vi "Cowl_Hardware_Begin.vi"(8 "error in":errorcluster) -> (0 "error out":errorcluster)   [LabVIEW 2020]
uses:
  <vilib>/Rock Robotics/WPI/ThirdParty/Phoenix-LabVIEW/Motor Controller/Controls/CTRE_Phoenix_MotorControl_NeutralMode.ctl
  <vilib>/Rock Robotics/WPI/ThirdParty/Phoenix-LabVIEW/Motor Controller/Controls/CTRE_Phoenix_MotorControl_SupplyCurrentLimitConfiguration.ctl
  Cowl_Hardware_Globals.vi
  <vilib>/Rock Robotics/WPI/ThirdParty/Phoenix-LabVIEW/Motor Controller/Controls/CTRE_Phoenix_MotorControl_StatusFrameEnhanced.ctl
panel:
  out "appended array":u32[](array[numeric])
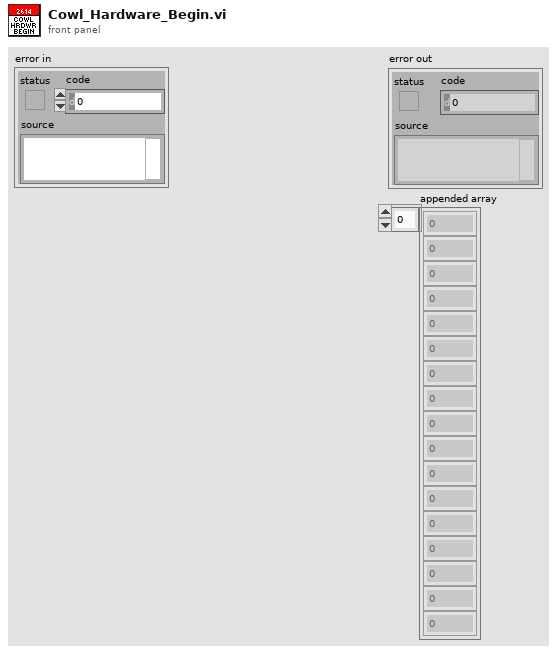
[diagram p1: front panel]
types:
  T1 = typedef "CTRE_Phoenix_MotorControl_SupplyCurrentLimitConfiguration.ctl" = cluster{"Enable?":bool, "Current Limit":dbl, "Threshold Current":dbl, "Threshold Time":dbl}
  T2 = typedef "CTRE_Phoenix_MotorControl_NeutralMode.ctl" = enum8{"EEPROMSetting", "Override to Coast", "Override to Brake"}
  T3 = typedef "WPI_MotorControlDeviceRef.ctl" = cluster{"DeviceStatus":errorcluster, "Type":T4, "PWM":cluster{"PWM Channel":T5, "DeadBand":T6}, "CAN":cluster{"Device Number":u8, "SetOutput VI Ref":variant, "GetOutput VI Ref":variant, "Enable VI Ref":variant, "Disable VI Ref":variant, "Data":variant}, "Invert":bool, "DIO PWM":cluster{"PWM \"Enable\" Channel":T5, "DIOChannel":T7, "PWM Rate":dbl}}
  T4 = typedef "WPI_MotorControlType.ctl" = enum16{"PWM", "CAN", "DIO PWM"}
  T5 = typedef "FPGA_DIOPWMChannel.ctl" = enum8{"PWM 0", "PWM 1", "PWM 2", "PWM 3", "PWM 4", "PWM 5", "PWM 6", "PWM 7", "PWM 8", "PWM 9", "PWM MXP 0", "PWM MXP 1", "PWM MXP 2", "PWM MXP 3", "PWM MXP 4", "PWM MXP 5", "PWM MXP 6", "PWM MXP 7", "PWM MXP 8", "PWM MXP 9", "Invalid"}
  T6 = typedef "WPI_PWMDeadband.ctl" = cluster{"Name":string, "maxPositivePwm":i32, "minPositivePwm":i32, "centerPwm":i32, "maxNegativePwm":i32, "minNegativePwm":i32, "angularRange":u16}
  T7 = typedef "FPGA_DIOChannel.ctl" = enum8{"DIO 0", "DIO 1", "DIO 2", "DIO 3", "DIO 4", "DIO 5", "DIO 6", "DIO 7", "DIO 8", "DIO 9", "DIO MXP 0", "DIO MXP 1", "DIO MXP 2", "DIO MXP 3", "DIO MXP 4", "DIO MXP 5", "DIO MXP 6", "DIO MXP 7", "DIO MXP 8", "DIO MXP 9", "DIO MXP 10", "DIO MXP 11", "DIO MXP 12", "DIO MXP 13", "DIO MXP 14", "DIO MXP 15", "SPI Port CS1", "SPI Port CS2", "SPI Port CS3", "SPI Port MISO", "SPI Port MOSI", "Invalid"}
  T8 = typedef "CTRE_Phoenix_MotorControl_StatusFrameEnhanced.ctl" = u16
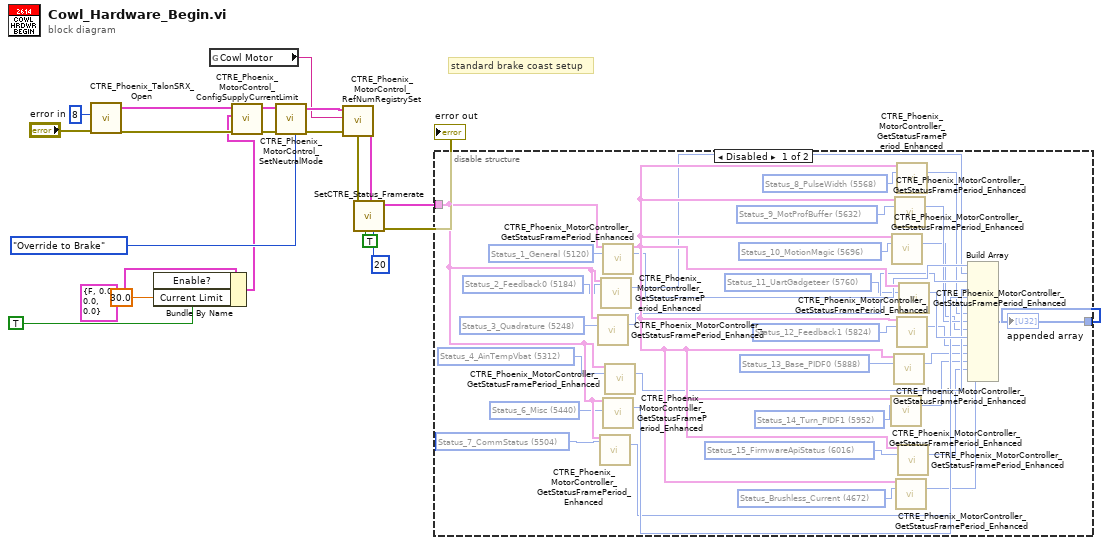
[diagram p0: block diagram]
diagram:
  # "standard brake coast setup"
  n1 = call <vilib>:"CTRE_Phoenix_TalonSRX_Open.vi"("error in"="error in", "Device Number"=u8 8) -> ("error out"=w17:errorcluster, "PhoenixMotorControlDevRef"=w18:T3)  [unwired: 8 in]
  n2 = Bundle By Name(cluster=T1 {"Enable?"=FALSE, "Current Limit"=0.0, "Threshold Current"=0.0, "Threshold Time"=0.0} ("Supply Current Limit Configuration"), "Enable?"=TRUE, "Current Limit"=30.0) -> (w10:T1)
  n3 = global read "Cowl_Hardware_Globals.vi" "Cowl Motor"() -> (w9:string)
  n4 = call <vilib>:"CTRE_Phoenix_MotorControl_ConfigSupplyCurrentLimit.vi"("error in (no error)"=w17, "Supply Current Limit Configuration"=w10, "PhoenixMotorControlDevRef"=w18) -> ("error out"=w16:errorcluster, "PhoenixMotorControlDevRef"=w15:T3)  [unwired: 7 in]
  n5 = call <vilib>:"CTRE_Phoenix_MotorControl_SetNeutralMode.vi"("error in (no error)"=w16, "Motor Control Neutral Mode"=CTRE_Phoenix_MotorControl_NeutralMode."Override to Brake", "PhoenixMotorControlDevRef"=w15) -> ("error out"=w14:errorcluster, "PhoenixMotorControlDevRef"=w19:T3)  [unwired: 7 in]
  n6 = call <vilib>:"CTRE_Phoenix_MotorControl_RefNumRegistrySet.vi"("error in (no error)"=w14, "refnum name"=w9, "PhoenixMotorControlDevRef"=w19) -> ("error out"=w6:errorcluster, "PhoenixMotorControlDevRef"=w7:T3)  [unwired: 7 in]
  n7 = call "SetCTRE_Status_Framerate.vi"("STATUS2Override(ms)"=20, "STATUS2OutsideOverride"=TRUE, "error in (no error)"=w6, "PhoenixMotorControlDevRef"=w7) -> ("error out"=→"error out":errorcluster, "PhoenixMotorControlDevRef 2"=w1:T3)  [unwired: 6 in]
  n8 = disable-structure shown="Disabled" {
    disable-tunnel: w1 -> [w50 _]
    disable-tunnel: [w54 _] -> w2
    frame Disabled {
      w22 = T8 5760 items=["Status_1_General"=5120, "Status_2_Feedback0"=5184, "Status_3_Quadrature"=5248, "Status_4_AinTempVbat"=5312, "Status_6_Misc"=5440, "Status_7_CommStatus"=5504, "Status_8_PulseWidth"=5568, "Status_9_MotProfBuffer"=5632, "Status_10_MotionMagic"=5696, "Status_11_UartGadgeteer"=5760, "Status_12_Feedback1"=5824, "Status_13_Base_PIDF0"=5888, "Status_14_Turn_PIDF1"=5952, "Status_15_FirmwareApiStatus"=6016, "Status_Brushless_Current"=4672] ("Status Frame")
      w23 = T8 5696 items=["Status_1_General"=5120, "Status_2_Feedback0"=5184, "Status_3_Quadrature"=5248, "Status_4_AinTempVbat"=5312, "Status_6_Misc"=5440, "Status_7_CommStatus"=5504, "Status_8_PulseWidth"=5568, "Status_9_MotProfBuffer"=5632, "Status_10_MotionMagic"=5696, "Status_11_UartGadgeteer"=5760, "Status_12_Feedback1"=5824, "Status_13_Base_PIDF0"=5888, "Status_14_Turn_PIDF1"=5952, "Status_15_FirmwareApiStatus"=6016, "Status_Brushless_Current"=4672] ("Status Frame")
      w25 = T8 5888 items=["Status_1_General"=5120, "Status_2_Feedback0"=5184, "Status_3_Quadrature"=5248, "Status_4_AinTempVbat"=5312, "Status_6_Misc"=5440, "Status_7_CommStatus"=5504, "Status_8_PulseWidth"=5568, "Status_9_MotProfBuffer"=5632, "Status_10_MotionMagic"=5696, "Status_11_UartGadgeteer"=5760, "Status_12_Feedback1"=5824, "Status_13_Base_PIDF0"=5888, "Status_14_Turn_PIDF1"=5952, "Status_15_FirmwareApiStatus"=6016, "Status_Brushless_Current"=4672] ("Status Frame")
      w27 = T8 6016 items=["Status_1_General"=5120, "Status_2_Feedback0"=5184, "Status_3_Quadrature"=5248, "Status_4_AinTempVbat"=5312, "Status_6_Misc"=5440, "Status_7_CommStatus"=5504, "Status_8_PulseWidth"=5568, "Status_9_MotProfBuffer"=5632, "Status_10_MotionMagic"=5696, "Status_11_UartGadgeteer"=5760, "Status_12_Feedback1"=5824, "Status_13_Base_PIDF0"=5888, "Status_14_Turn_PIDF1"=5952, "Status_15_FirmwareApiStatus"=6016, "Status_Brushless_Current"=4672] ("Status Frame")
      w29 = T8 5952 items=["Status_1_General"=5120, "Status_2_Feedback0"=5184, "Status_3_Quadrature"=5248, "Status_4_AinTempVbat"=5312, "Status_6_Misc"=5440, "Status_7_CommStatus"=5504, "Status_8_PulseWidth"=5568, "Status_9_MotProfBuffer"=5632, "Status_10_MotionMagic"=5696, "Status_11_UartGadgeteer"=5760, "Status_12_Feedback1"=5824, "Status_13_Base_PIDF0"=5888, "Status_14_Turn_PIDF1"=5952, "Status_15_FirmwareApiStatus"=6016, "Status_Brushless_Current"=4672] ("Status Frame")
      w31 = T8 5568 items=["Status_1_General"=5120, "Status_2_Feedback0"=5184, "Status_3_Quadrature"=5248, "Status_4_AinTempVbat"=5312, "Status_6_Misc"=5440, "Status_7_CommStatus"=5504, "Status_8_PulseWidth"=5568, "Status_9_MotProfBuffer"=5632, "Status_10_MotionMagic"=5696, "Status_11_UartGadgeteer"=5760, "Status_12_Feedback1"=5824, "Status_13_Base_PIDF0"=5888, "Status_14_Turn_PIDF1"=5952, "Status_15_FirmwareApiStatus"=6016, "Status_Brushless_Current"=4672] ("Status Frame")
      w33 = T8 4672 items=["Status_1_General"=5120, "Status_2_Feedback0"=5184, "Status_3_Quadrature"=5248, "Status_4_AinTempVbat"=5312, "Status_6_Misc"=5440, "Status_7_CommStatus"=5504, "Status_8_PulseWidth"=5568, "Status_9_MotProfBuffer"=5632, "Status_10_MotionMagic"=5696, "Status_11_UartGadgeteer"=5760, "Status_12_Feedback1"=5824, "Status_13_Base_PIDF0"=5888, "Status_14_Turn_PIDF1"=5952, "Status_15_FirmwareApiStatus"=6016, "Status_Brushless_Current"=4672] ("Status Frame")
      w35 = T8 5824 items=["Status_1_General"=5120, "Status_2_Feedback0"=5184, "Status_3_Quadrature"=5248, "Status_4_AinTempVbat"=5312, "Status_6_Misc"=5440, "Status_7_CommStatus"=5504, "Status_8_PulseWidth"=5568, "Status_9_MotProfBuffer"=5632, "Status_10_MotionMagic"=5696, "Status_11_UartGadgeteer"=5760, "Status_12_Feedback1"=5824, "Status_13_Base_PIDF0"=5888, "Status_14_Turn_PIDF1"=5952, "Status_15_FirmwareApiStatus"=6016, "Status_Brushless_Current"=4672] ("Status Frame")
      w37 = T8 5632 items=["Status_1_General"=5120, "Status_2_Feedback0"=5184, "Status_3_Quadrature"=5248, "Status_4_AinTempVbat"=5312, "Status_6_Misc"=5440, "Status_7_CommStatus"=5504, "Status_8_PulseWidth"=5568, "Status_9_MotProfBuffer"=5632, "Status_10_MotionMagic"=5696, "Status_11_UartGadgeteer"=5760, "Status_12_Feedback1"=5824, "Status_13_Base_PIDF0"=5888, "Status_14_Turn_PIDF1"=5952, "Status_15_FirmwareApiStatus"=6016, "Status_Brushless_Current"=4672] ("Status Frame")
      w39 = T8 5120 items=["Status_1_General"=5120, "Status_2_Feedback0"=5184, "Status_3_Quadrature"=5248, "Status_4_AinTempVbat"=5312, "Status_6_Misc"=5440, "Status_7_CommStatus"=5504, "Status_8_PulseWidth"=5568, "Status_9_MotProfBuffer"=5632, "Status_10_MotionMagic"=5696, "Status_11_UartGadgeteer"=5760, "Status_12_Feedback1"=5824, "Status_13_Base_PIDF0"=5888, "Status_14_Turn_PIDF1"=5952, "Status_15_FirmwareApiStatus"=6016, "Status_Brushless_Current"=4672] ("Status Frame")
      w40 = T8 5504 items=["Status_1_General"=5120, "Status_2_Feedback0"=5184, "Status_3_Quadrature"=5248, "Status_4_AinTempVbat"=5312, "Status_6_Misc"=5440, "Status_7_CommStatus"=5504, "Status_8_PulseWidth"=5568, "Status_9_MotProfBuffer"=5632, "Status_10_MotionMagic"=5696, "Status_11_UartGadgeteer"=5760, "Status_12_Feedback1"=5824, "Status_13_Base_PIDF0"=5888, "Status_14_Turn_PIDF1"=5952, "Status_15_FirmwareApiStatus"=6016, "Status_Brushless_Current"=4672] ("Status Frame")
      w42 = T8 5184 items=["Status_1_General"=5120, "Status_2_Feedback0"=5184, "Status_3_Quadrature"=5248, "Status_4_AinTempVbat"=5312, "Status_6_Misc"=5440, "Status_7_CommStatus"=5504, "Status_8_PulseWidth"=5568, "Status_9_MotProfBuffer"=5632, "Status_10_MotionMagic"=5696, "Status_11_UartGadgeteer"=5760, "Status_12_Feedback1"=5824, "Status_13_Base_PIDF0"=5888, "Status_14_Turn_PIDF1"=5952, "Status_15_FirmwareApiStatus"=6016, "Status_Brushless_Current"=4672] ("Status Frame")
      w44 = T8 5440 items=["Status_1_General"=5120, "Status_2_Feedback0"=5184, "Status_3_Quadrature"=5248, "Status_4_AinTempVbat"=5312, "Status_6_Misc"=5440, "Status_7_CommStatus"=5504, "Status_8_PulseWidth"=5568, "Status_9_MotProfBuffer"=5632, "Status_10_MotionMagic"=5696, "Status_11_UartGadgeteer"=5760, "Status_12_Feedback1"=5824, "Status_13_Base_PIDF0"=5888, "Status_14_Turn_PIDF1"=5952, "Status_15_FirmwareApiStatus"=6016, "Status_Brushless_Current"=4672] ("Status Frame")
      w46 = T8 5248 items=["Status_1_General"=5120, "Status_2_Feedback0"=5184, "Status_3_Quadrature"=5248, "Status_4_AinTempVbat"=5312, "Status_6_Misc"=5440, "Status_7_CommStatus"=5504, "Status_8_PulseWidth"=5568, "Status_9_MotProfBuffer"=5632, "Status_10_MotionMagic"=5696, "Status_11_UartGadgeteer"=5760, "Status_12_Feedback1"=5824, "Status_13_Base_PIDF0"=5888, "Status_14_Turn_PIDF1"=5952, "Status_15_FirmwareApiStatus"=6016, "Status_Brushless_Current"=4672] ("Status Frame")
      w48 = T8 5312 items=["Status_1_General"=5120, "Status_2_Feedback0"=5184, "Status_3_Quadrature"=5248, "Status_4_AinTempVbat"=5312, "Status_6_Misc"=5440, "Status_7_CommStatus"=5504, "Status_8_PulseWidth"=5568, "Status_9_MotProfBuffer"=5632, "Status_10_MotionMagic"=5696, "Status_11_UartGadgeteer"=5760, "Status_12_Feedback1"=5824, "Status_13_Base_PIDF0"=5888, "Status_14_Turn_PIDF1"=5952, "Status_15_FirmwareApiStatus"=6016, "Status_Brushless_Current"=4672] ("Status Frame")
      n9 = call <vilib>:"CTRE_Phoenix_MotorController_GetStatusFramePeriod_Enhanced.vi"("PhoenixMotorControlDevRef"=w50, "Status Frame"=w46) -> ("periodMs"=w47:u32)  [unwired: 11 in, 2 out]
      n10 = call <vilib>:"CTRE_Phoenix_MotorController_GetStatusFramePeriod_Enhanced.vi"("PhoenixMotorControlDevRef"=w50, "Status Frame"=w40) -> ("periodMs"=w41:u32)  [unwired: 11 in, 2 out]
      n11 = call <vilib>:"CTRE_Phoenix_MotorController_GetStatusFramePeriod_Enhanced.vi"("PhoenixMotorControlDevRef"=w50, "Status Frame"=w42) -> ("periodMs"=w43:u32)  [unwired: 11 in, 2 out]
      n12 = call <vilib>:"CTRE_Phoenix_MotorController_GetStatusFramePeriod_Enhanced.vi"("PhoenixMotorControlDevRef"=w50, "Status Frame"=w39) -> ("PhoenixMotorControlDevRef"=w52:T3, "periodMs"=w51:u32)  [unwired: 11 in, 1 out]
      n13 = call <vilib>:"CTRE_Phoenix_MotorController_GetStatusFramePeriod_Enhanced.vi"("PhoenixMotorControlDevRef"=w50, "Status Frame"=w44) -> ("periodMs"=w45:u32)  [unwired: 11 in, 2 out]
      n14 = call <vilib>:"CTRE_Phoenix_MotorController_GetStatusFramePeriod_Enhanced.vi"("PhoenixMotorControlDevRef"=w50, "Status Frame"=w48) -> ("periodMs"=w49:u32)  [unwired: 11 in, 2 out]
      n15 = call <vilib>:"CTRE_Phoenix_MotorController_GetStatusFramePeriod_Enhanced.vi"("PhoenixMotorControlDevRef"=w52, "Status Frame"=w29) -> ("periodMs"=w30:u32)  [unwired: 11 in, 2 out]
      n16 = call <vilib>:"CTRE_Phoenix_MotorController_GetStatusFramePeriod_Enhanced.vi"("PhoenixMotorControlDevRef"=w52, "Status Frame"=w23) -> ("periodMs"=w24:u32)  [unwired: 11 in, 2 out]
      n17 = call <vilib>:"CTRE_Phoenix_MotorController_GetStatusFramePeriod_Enhanced.vi"("PhoenixMotorControlDevRef"=w52, "Status Frame"=w25) -> ("periodMs"=w26:u32)  [unwired: 11 in, 2 out]
      n18 = call <vilib>:"CTRE_Phoenix_MotorController_GetStatusFramePeriod_Enhanced.vi"("PhoenixMotorControlDevRef"=w52, "Status Frame"=w37) -> ("periodMs"=w38:u32)  [unwired: 11 in, 2 out]
      n19 = call <vilib>:"CTRE_Phoenix_MotorController_GetStatusFramePeriod_Enhanced.vi"("PhoenixMotorControlDevRef"=w52, "Status Frame"=w33) -> ("periodMs"=w34:u32)  [unwired: 11 in, 2 out]
      n20 = call <vilib>:"CTRE_Phoenix_MotorController_GetStatusFramePeriod_Enhanced.vi"("PhoenixMotorControlDevRef"=w52, "Status Frame"=w31) -> ("periodMs"=w32:u32)  [unwired: 11 in, 2 out]
      n21 = call <vilib>:"CTRE_Phoenix_MotorController_GetStatusFramePeriod_Enhanced.vi"("PhoenixMotorControlDevRef"=w52, "Status Frame"=w35) -> ("periodMs"=w36:u32)  [unwired: 11 in, 2 out]
      n22 = call <vilib>:"CTRE_Phoenix_MotorController_GetStatusFramePeriod_Enhanced.vi"("PhoenixMotorControlDevRef"=w52, "Status Frame"=w27) -> ("periodMs"=w28:u32)  [unwired: 11 in, 2 out]
      n23 = call <vilib>:"CTRE_Phoenix_MotorController_GetStatusFramePeriod_Enhanced.vi"("PhoenixMotorControlDevRef"=w52, "Status Frame"=w22) -> ("periodMs"=w53:u32)  [unwired: 11 in, 2 out]
      n24 = Build Array(w51, w43, w47, w49, w45, w41, w32, w38, w24, w53, w36, w26, w30, w28, w34) -> (w54:u32[])
    }
    frame Enabled {
    }
  }
  "appended array" <- w2
